vi "GVProbenvol.vi"() -> ()   [LabVIEW 2017]
panel:
  out "Probenvol.2":dbl
  out "Probenvol.1":dbl
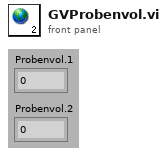
[diagram p1: front panel]
diagram:
